vi "GV_CalcIncrement.vi"(0 "FormatString":string, 1 "desired font(Application)":T4(ring)=enum."Application Font", 2 "scale definition":T1={"coordinate 1"=5, "value 1"=5.0, "coordinate 2"=5, "value 2"=5.0, "log?(F)"=FALSE} {"value 2" format="%0.2f"; "value 1" format="%0.2f"}, 3 "scale attributes":T2={"horizontal"=TRUE, "left/top"=FALSE, "draw bar"=FALSE, "line color"=0, "text color"=0}, 5 "[user-specified font]":T3) -> (6 "start":dbl format="%0.2f", 7 "increment":dbl format="%0.2f", 9 "text size":i16)   [LabVIEW 2020, in "Sgraph_lib_V1.lvlib" / "Gviewer.lvclass"]
uses:
  Gviewer.lvclass
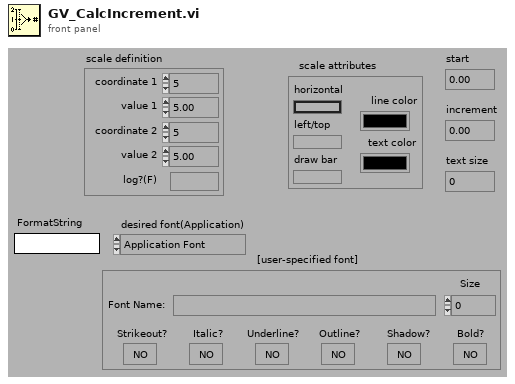
[diagram p1: front panel]
types:
  T1 = cluster{"coordinate 1":i16, "value 1":dbl, "coordinate 2":i16, "value 2":dbl, "log?(F)":bool}
  T2 = cluster{"horizontal":bool, "left/top":bool, "draw bar":bool, "line color":u32, "text color":u32}
  T3 = cluster{"Font Name:":string, "Size":i16, "Strikeout?":bool, "Italic?":bool, "Underline?":bool, "Outline?":bool, "Shadow?":bool, "Bold?":bool}
  T4 = enum16{"User-specified Font", "Application Font", "System Font", "Dialog Font"}
  T5 = cluster{"left":i16, "top":i16, "right":i16, "bottom":i16}
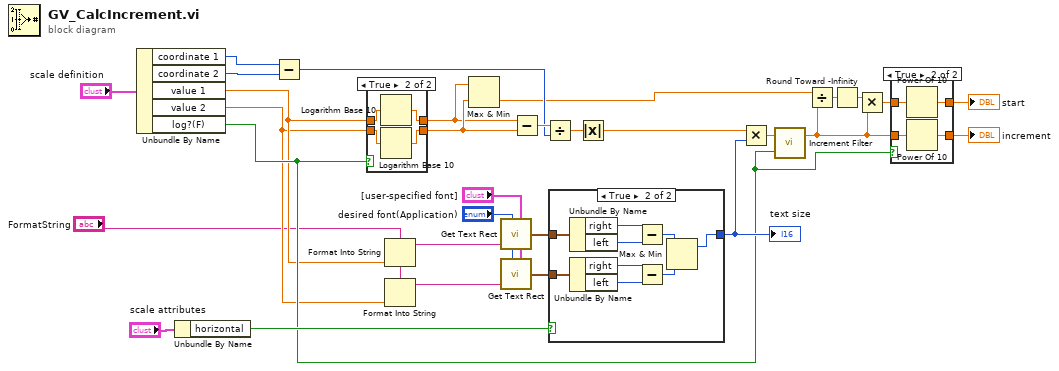
[diagram p0: block diagram]
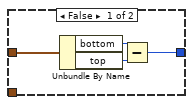
[diagram p4: hidden frame]
diagram:
  n1 = Unbundle By Name("scale definition") -> ("coordinate 1"=w17:i16, "coordinate 2"=w18:i16, "value 1"=w5:dbl, "value 2"=w4:dbl, "log?(F)"=w6:bool)
  n2 = Unbundle By Name("scale attributes") -> ("horizontal"=w26:bool)
  n3 = Subtract(x=w17, y=w18) -> (x-y=w19:i16)
  n4 = case shown="True" w6 {
    tunnel: w5 -> [w32 w35]
    tunnel: [w32 w34] -> w13
    tunnel: w4 -> [w31 w36]
    tunnel: [w31 w33] -> w14
    frame False {
    }
    frame True {
      n5 = Logarithm Base 10(1:w35) -> (0:w34:dbl)
      n6 = Logarithm Base 10(1:w36) -> (0:w33:dbl)
    }
  }
  n7 = Format Into String(format string="FormatString", w5) -> (resulting string=w2:string)  [unwired: 2 in, 1 out]
  n8 = Format Into String(format string="FormatString", w4) -> (resulting string=w1:string)  [unwired: 2 in, 1 out]
  n9 = Max & Min(x=w13, y=w14) -> (min(x,y)=w12:dbl)  [unwired: 1 out]
  n10 = call <vilib>:"Get Text Rect.vi"("desired font(Application)"="desired font(Application)", "text"=w2, "[user-specified font]"="[user-specified font]") -> ("rect"=w24:T5)  [unwired: 6 in]
  n11 = call <vilib>:"Get Text Rect.vi"("desired font(Application)"="desired font(Application)", "text"=w1, "[user-specified font]"="[user-specified font]") -> ("rect"=w25:T5)  [unwired: 6 in]
  n12 = Subtract(x=w13, y=w14) -> (x-y=w21:dbl)
  n13 = Divide(x=w21, y=w19) -> (x/y=w23:dbl)
  n14 = case shown="True" w26 {
    tunnel: w25 -> [_ w48]
    tunnel: w24 -> [w38 w49]
    tunnel: [w37 w41] -> w20
    frame False {
      n15 = Unbundle By Name(w38) -> ("bottom"=w39:i16, "top"=w40:i16)
      n16 = Subtract(x=w39, y=w40) -> (x-y=w37:i16)
    }
    frame True {
      n17 = Unbundle By Name(w49) -> ("right"=w44:i16, "left"=w45:i16)
      n18 = Unbundle By Name(w48) -> ("right"=w47:i16, "left"=w46:i16)
      n19 = Subtract(x=w44, y=w45) -> (x-y=w42:i16)
      n20 = Subtract(x=w47, y=w46) -> (x-y=w43:i16)
      n21 = Max & Min(x=w42, y=w43) -> (max(x,y)=w41:i16)  [unwired: 1 out]
    }
  }
  "text size" <- w20
  n22 = Absolute Value(x=w23) -> (abs(x)=w22:dbl)
  n23 = Multiply(x=w22, y=w20) -> (x*y=w7:dbl)
  n24 = call <vilib>:"Increment Filter.vi"("log?(F)"=w6, "initial increment"=w7) -> ("nice increment"=w10:dbl)  [unwired: 1 in]
  n25 = Divide(x=w12, y=w10) -> (x/y=w16:dbl)
  n26 = Round Toward -Infinity(1:w16) -> (0:w15:dbl)
  n27 = Multiply(x=w15, y=w10) -> (x*y=w9:dbl)
  n28 = case shown="True" w6 {
    tunnel: w10 -> [w51 w55]
    tunnel: [w51 w54] -> w11
    tunnel: w9 -> [w50 w53]
    tunnel: [w50 w52] -> w8
    frame False {
    }
    frame True {
      n29 = Power Of 10(x=w53) -> (10^x=w52:dbl)
      n30 = Power Of 10(x=w55) -> (10^x=w54:dbl)
    }
  }
  "increment" <- w11
  "start" <- w8
